vi "create empty configuration.vi"(8 "error in (no error)":errorcluster) -> (0 "error out":errorcluster, 3 "DSFConfiguration out":refnum<class "DSFConfiguration.lvclass">)   [LabVIEW 2017, in "DSFConfiguration.lvclass"]
uses:
  DSFConfiguration.lvclass
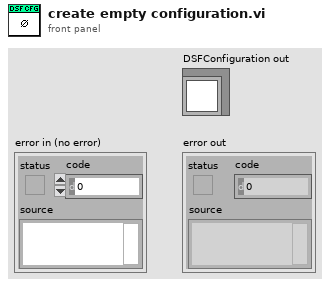
[diagram p1: front panel]
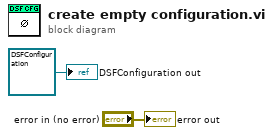
[diagram p0: block diagram]
diagram:
  "error out" <- "error in (no error)"
  "DSFConfiguration out" <- refnum<class "DSFConfiguration.lvclass"> refnum ("DSFConfiguration in")
